vi "AM Tx.vi"() -> ()   [LabVIEW 2011]
uses:
  <vilib>/sound2/lvsound2.llb/Sound Data Format.ctl
  <vilib>/sound2/lvsound2.llb/Sampling Mode.ctl
  <vilib>/sound2/lvsound2.llb/Sound Input Read (DBL).vi
  <vilib>/sound2/lvsound2.llb/Sound Output Write (DBL).vi
  <vilib>/addons/Modulation/Analog/MT Modulate AM (DSB).vi
  <instrlib>/niUSRP/niUSRP Write Tx Data (CDB Cluster).vi
  <vilib>/addons/Modulation/niAMT.lvlib
panel:
  out "Waveform Graph":waveform(dbl)(graph)
  in  "modulation index":dbl=1.0 format="%.2f"
  in  "Sound Format":T1={"sample rate (S/s)"=22050.0, "number of channels"=2, "bits per sample"=16}
  out "coerced gain":dbl format="%#_6f"
  in  "device names":refnum<k15>="192.168.10.2"
  in  "active antenna":string="TX1"
  in  "Capture Time (sec)":i32=10000
  in  "timeout":dbl=10.0
  out "error out":errorcluster
  in  "stop":bool
  out "coerced carrier frequency":dbl=100000.0 format="%#_6p"
  out "coerced IQ rate":dbl=100000.0 format="%#_6p"
  in  "gain":dbl format="%#_6f"
  in  "carrier frequency":dbl=2000000000.0 format="%#_6p"
  in  "IQ rate":dbl=10000000.0 format="%#_6p"
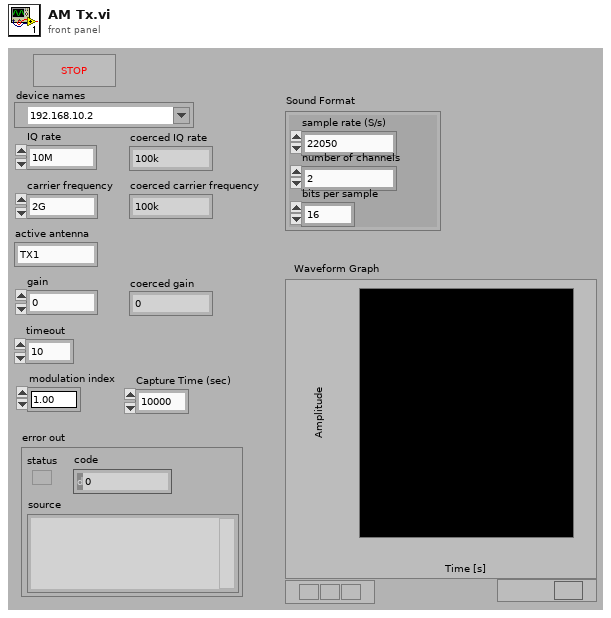
[diagram p1: front panel]
types:
  T1 = typedef "Sound Data Format.ctl" = cluster{"sample rate (S/s)":dbl, "number of channels":i32, "bits per sample":i32}
  T2 = typedef "Sampling Mode.ctl" = i32
  T3 = typedef "Sound Input Task ID.ctl" = u32
  T4 = typedef "Sound Output Task ID.ctl" = u32
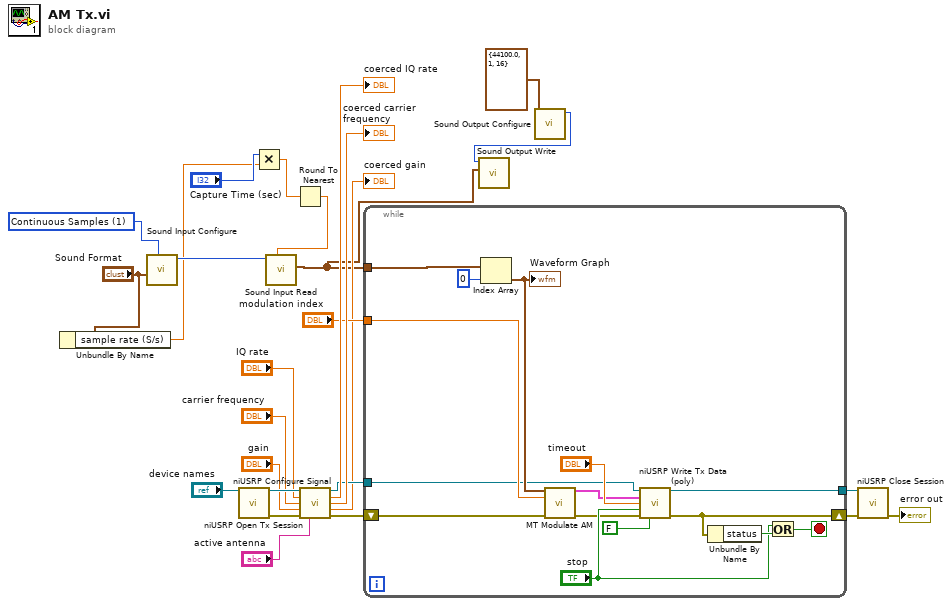
[diagram p0: block diagram]
diagram:
  w15 = T2 1 items=["Finite Samples", "Continuous Samples"] ("sample mode")
  n1 = Unbundle By Name("Sound Format") -> ("sample rate (S/s)"=w6:dbl)
  n2 = call <vilib>:"Sound Input Configure.vi"("sample mode"=w15, "sound format"="Sound Format") -> ("task ID"=w10:T3)  [unwired: 8 in, 1 out]
  n3 = call <instrlib>:"niUSRP Open Tx Session.vi"("device names"="device names") -> ("session handle out"=w25:refnum<k15>, "error out"=w23:errorcluster)  [unwired: 13 in]
  n4 = Multiply(x="Capture Time (sec)", y=w6) -> (x*y=w5:dbl)
  n5 = Round To Nearest(number=w5) -> (nearest integer value=w4:dbl)
  n6 = call-poly <vilib>:"Sound Input Read.vi"("number of samples/ch"=w4, "task ID"=w10) -> ("data"=w3:waveform(dbl)[])  [unwired: 7 in, 2 out]
  n7 = call <instrlib>:"niUSRP Configure Signal.vi"("session handle"=w25, "IQ rate"="IQ rate", "carrier frequency"="carrier frequency", "gain"="gain", "error in (no error)"=w23, "active antenna"="active antenna") -> ("session handle out"=w11:refnum<k15>, "coerced IQ rate"=→"coerced IQ rate":dbl, "coerced carrier frequency"=→"coerced carrier frequency":dbl, "coerced gain"=→"coerced gain":dbl, "error out"=w12:errorcluster)  [unwired: 5 in]
  n8 = while {
    tunnel: [w39] -> w21
    shift-right: [w38] -> w20
    shift-left: w12 -> [w30]
    tunnel: "modulation index" -> [w32]
    tunnel: w11 -> [w28]
    tunnel: w3 -> [w27]
    stop <- w41 stop-if-true
    n9 = Index Array(array=w27, index=0) -> (element=w31:waveform(dbl))
    "Waveform Graph" <- w31
    n10 = call-poly <vilib>:"MT Modulate AM.vi"("message signal"=w31, "modulation index"=w32, "error in (no error)"=w30) -> ("AM modulated waveform"=w35:cluster{"t0":dbl, "dt":dbl, "Y":cdb[]}, "error out"=w34:errorcluster)  [unwired: 11 in]
    n11 = call-poly <instrlib>:"niUSRP Write Tx Data (poly).vi"("session handle"=w28, "data"=w35, "timeout"="timeout", "end of data?"="stop", "error in (no error)"=w34, "use waveform dt for IQ rate?"=FALSE) -> ("session handle out"=w39:refnum<k15>, "error out"=w38:errorcluster)  [unwired: 8 in]
    n12 = Unbundle By Name(w38) -> ("status"=w37:bool)
    n13 = Or(x="stop", y=w37) -> (x .or. y?=w41:bool)
  }
  n14 = call <vilib>:"Sound Output Configure.vi"("sound format"=T1 {"sample rate (S/s)"=44100.0, "number of channels"=1, "bits per sample"=16}) -> ("task ID"=w2:T4)  [unwired: 9 in, 1 out]
  n15 = call-poly <vilib>:"Sound Output Write.vi"("data"=w3, "task ID"=w2) -> ()  [unwired: 8 in, 2 out]
  n16 = call <instrlib>:"niUSRP Close Session.vi"("session handle"=w21, "error in (no error)"=w20) -> ("error out"=→"error out":errorcluster)  [unwired: 13 in]
